vi "hydraharp_set_sync_settings.vi"(8 "error in (no error)":errorcluster, 10 "sync_settings":T1 {"snc_offs" min=-99999 max=99999 step=1; "snc_ZeroX" min=0 max=20 step=1; "snc_level" min=0 max=800 step=10}, 11 "hydraharp in":refnum<class "hydraharp.lvclass">) -> (0 "error out":errorcluster, 3 "hydraharp out":refnum<class "hydraharp.lvclass">)   [LabVIEW 2015, in "hydraharp.lvclass"]
uses:
  hydraharp.lvclass
  hydraharp_panel/hpanel_sync_settings.ctl
  hydraharp_panel/hpanel_sync_div.ctl
  hydraharp.lvclass/hydraharp.ctl
  hhlib.dll
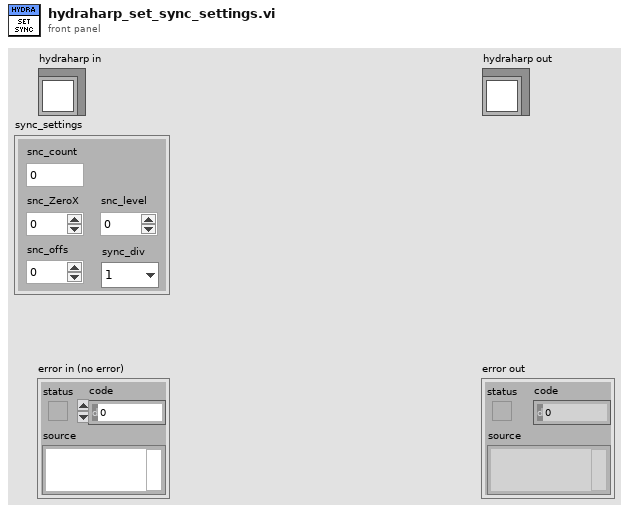
[diagram p1: front panel]
types:
  T1 = typedef "hpanel_sync_settings.ctl" = cluster{"snc_count":i32, "snc_level":i32, "snc_ZeroX":i32, "snc_offs":i32, "sync_div":T2}
  T2 = typedef "hpanel_sync_div.ctl" = enum16{"1", "2", "4", "8"}
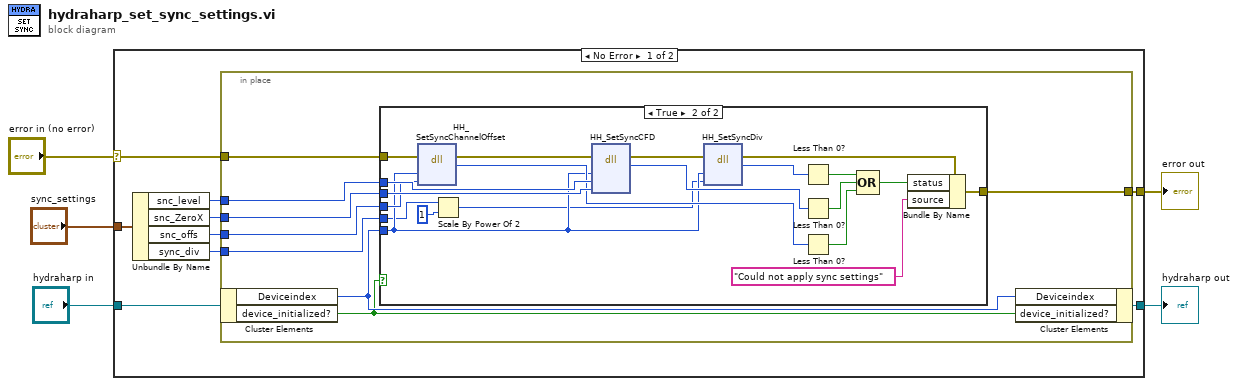
[diagram p0: block diagram]
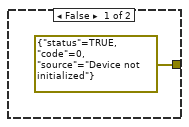
[diagram p2: hidden frame]
diagram:
  n1 = case shown="No Error" "error in (no error)" {
    selector: "error in (no error)" -> [w13 w45]
    tunnel: [w12 w45] -> w4
    tunnel: [w6 w44] -> w2
    tunnel: "hydraharp in" -> [w14 w44]
    tunnel: "sync_settings" -> [w11 _]
    frame No Error {
      n2 = Unbundle By Name(w11) -> ("snc_level"=w10:i32, "snc_ZeroX"=w9:i32, "snc_offs"=w7:i32, "sync_div"=w8:T2)
      n3 = in-place {
        in-place-border: w13 -> [w22]
        in-place-border: [w18] -> w12
        in-place-border: w10 -> [w21]
        in-place-border: w9 -> [w20]
        in-place-border: w8 -> [w16]
        in-place-border: w7 -> [w19]
        n4 = in-place-cluster #1(w14) -> ("Deviceindex"=w17:i32, "device_initialized?"=w15:bool)
        n5 = case shown="True" w15 {
          tunnel: w22 -> [_ w43]
          tunnel: w21 -> [_ w40]
          tunnel: w20 -> [_ w39]
          tunnel: w19 -> [_ w38]
          tunnel: [errorcluster {"status"=TRUE, "code"=0, "source"="Device not initialized"} ("error out") w24] -> w18
          tunnel: w17 -> [_ w31]
          tunnel: w16 -> [_ w29]
          frame False {
          }
          frame True {
            n6 = dll-call lib="hhlib.dll" fn="HH_SetSyncChannelOffset"(error in=w43, "devidx"=w31, "offset"=w38) -> (error out=w42:errorcluster, w37:i32)  [unwired: 4 in, 1 out]
            n7 = Scale By Power Of 2(n=w29, x=1) -> (x*2^n=w28:i32)
            n8 = dll-call lib="hhlib.dll" fn="HH_SetSyncCFD"(error in=w42, "devidx"=w31, "level"=w40, "zerox"=w39) -> (error out=w41:errorcluster, w36:i32)  [unwired: 5 in, 1 out]
            n9 = dll-call lib="hhlib.dll" fn="HH_SetSyncDiv"(error in=w41, "devidx"=w31, "divider"=w28) -> (error out=w27:errorcluster, w35:i32)  [unwired: 4 in, 1 out]
            n10 = Less Than 0?(x=w35) -> (x < 0?=w34:bool)
            n11 = Less Than 0?(x=w36) -> (x < 0?=w33:bool)
            n12 = Less Than 0?(x=w37) -> (x < 0?=w32:bool)
            n13 = Compound Arithmetic op=OR(w34, w33, w32) -> (w26:bool)
            n14 = Bundle By Name(cluster=w27, "status"=w26, "source"="Could not apply sync settings") -> (w24:errorcluster)
          }
        }
        n15 = in-place-cluster #1("Deviceindex"=w17, "device_initialized?"=w15) -> (w6:refnum<class "hydraharp.lvclass">)
      }
    }
    frame Error {
    }
  }
  "error out" <- w4
  "hydraharp out" <- w2
